vi "rawcdc_protocol.vi"() -> ()   [LabVIEW 2024]
doc: "This example performs writes and reads on a serial port, as directed by the user. You can press the Write and Read buttons, and change the Read Count, while the example is running.\n\nThe parameters set for the serial port must match the parameters of the connected instrument or device. In this example, the Read Count parameter specifies the number of bytes that the serial port reads. If there were more bytes at the port than the specified number, those bytes would not be read. If there were less bytes at the port than the specified number, you would receive a timeout error.\n\nThis example expands upon the flow control options for XON and XOFF, allowing the user to choose those control characters. Also, the user can enable or disable a termination character. Some devices require a termination character in order to identify the end of command strings. Some devices send a termination character to signify the end of data to be read. This example shows how you can end the Read operation once a termination character is detected in the buffer and/or append a termination character at the end of the Write data."
uses:
  <vilib>/Instr/_visa.llb/VISA Configure Serial Port (Instr).vi
panel:
  in  "Correction":dbl(slide) scale=-10.0..10.0
  out "Measured":dbl
  out "Waveform Chart":dbl[](graph)
  in  "Command List":string="stop\nencode 0\nslist 0 0\nsrate 6000\nps 2\ndec 1\ndeca 3\nnop\n\n\n"
  in  "Stop":bool
  in  "2108 CDC Virtual COM":refnum<visa-resource-name>="COM11"
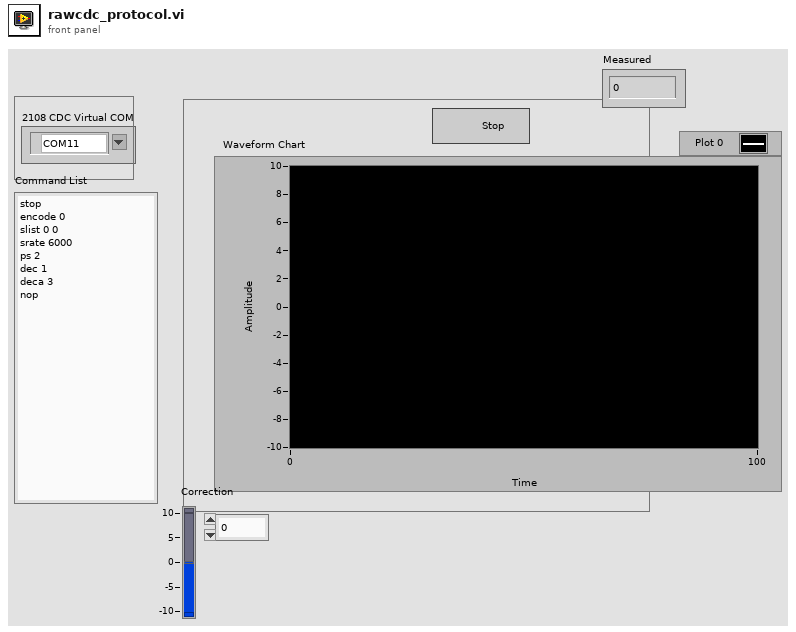
[diagram p1: front panel]
types:
  T1 = enum16{"big-endian, network order", "native, host order", "little-endian"}
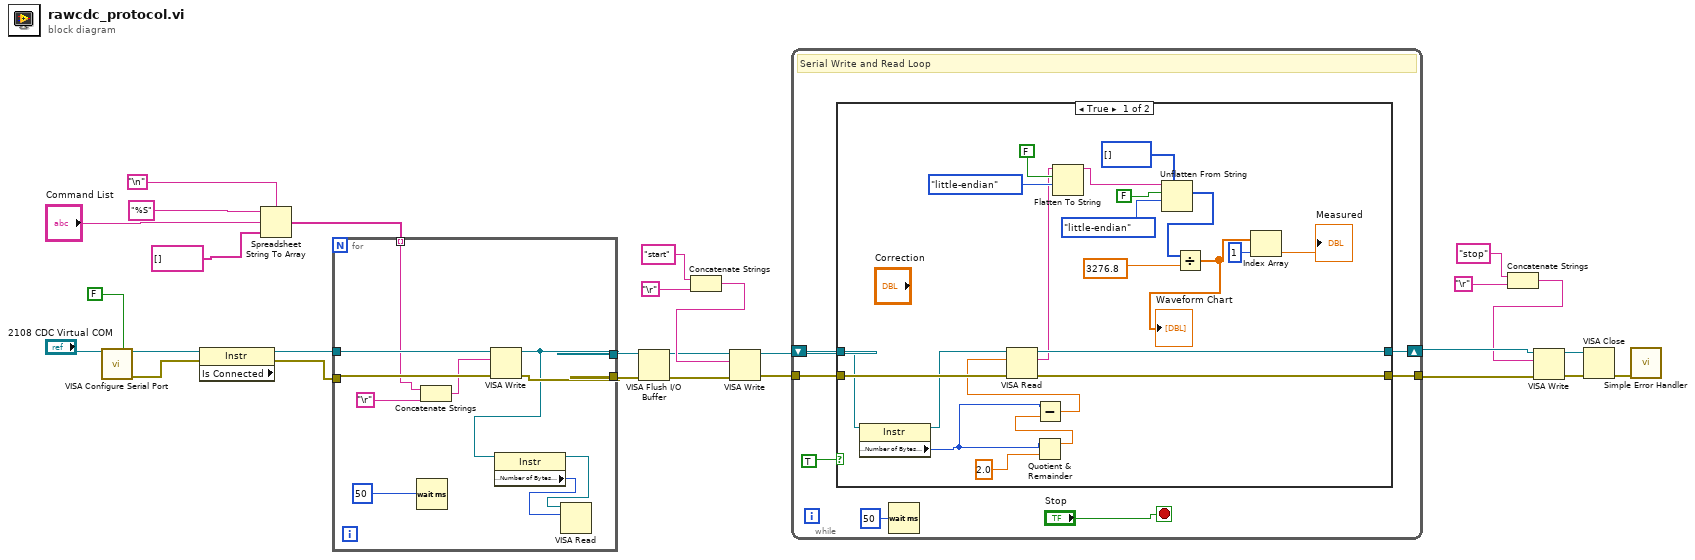
[diagram p0: block diagram]
diagram:
  n1 = call-poly "VISA Configure Serial Port"("VISA resource name"="2108 CDC Virtual COM", "Enable Termination\nChar (T)"=FALSE) -> ("VISA resource name out"=w26:refnum<visa-resource-name>, "error out"=w28:errorcluster)  [unwired: 8 in, 4 out]
  n2 = property class="Instr" props=["Is Connected"](reference=w26, error in=w28) -> (reference out=w2:refnum<visa-resource-name>, error out=w1:errorcluster)  [unwired: 1 out]
  n3 = Spreadsheet String To Array(delimiter (Tab)="\n", format string="%S", spreadsheet string="Command List", array type (2D Dbl)=string[] []) -> (array=w22:string[])
  n4 = for {
    tunnel: w22 -> [w35] mode=indexing
    tunnel: w2 -> [w38]
    tunnel: w1 -> [w37]
    tunnel: [w31] -> w6
    tunnel: [w32] -> w4
    n5 = Wait (ms)(milliseconds to wait=u32 50) -> ()  [unwired: 1 out]
    n6 = Concatenate Strings(w35, "\r") -> (w33:string)
    n7 = VISA Write(VISA resource name=w38, write buffer=w33, error in (no error)=w37) -> (VISA resource name out=w31:refnum<visa-resource-name>, error out=w32:errorcluster)  [unwired: 1 out]
    n8 = property class="Instr"(reference=w31) -> (reference out=w30:refnum<visa-resource-name>, "Serial Settings:Number of Bytes at Serial Port"=w29:u32)  [unwired: 1 in, 1 out]
    n9 = VISA Read(VISA resource name=w30, byte count=w29) -> ()  [unwired: 1 in, 4 out]
  }
  n10 = VISA Flush I/O Buffer(VISA resource name=w6, error in (no error)=w4) -> (VISA resource name out=w5:refnum<visa-resource-name>, error out=w3:errorcluster)  [unwired: 1 in]
  n11 = Concatenate Strings("start", "\r") -> (w10:string)
  n12 = VISA Write(VISA resource name=w5, write buffer=w10, error in (no error)=w3) -> (VISA resource name out=w9:refnum<visa-resource-name>, error out=w8:errorcluster)  [unwired: 1 out]
  n13 = while {
    shift-right: [w45] -> w19
    shift-left: w9 -> [w41]
    tunnel: w8 -> [w40]
    tunnel: [w43] -> w16
    stop <- "Stop" stop-if-true
    # "Serial Write and Read Loop"
    n14 = case shown="True" TRUE {
      tunnel: [w65 w68] -> w45
      tunnel: w41 -> [w63 w68]
      tunnel: w40 -> [w66 w67]
      tunnel: [w58 w67] -> w43
      frame True {
        n15 = property class="Instr"(reference=w63) -> (reference out=w57:refnum<visa-resource-name>, "Serial Settings:Number of Bytes at Serial Port"=w62:u32)  [unwired: 1 in, 1 out]
        n16 = Quotient & Remainder(x=w62, y=2.0) -> (x-y*floor(x/y)=w60:dbl)  [unwired: 1 out]
        n17 = Subtract(x=w62, y=w60) -> (x-y=w59:dbl)
        n18 = VISA Read(VISA resource name=w57, byte count=w59, error in (no error)=w66) -> (VISA resource name out=w65:refnum<visa-resource-name>, read buffer=w51:string, error out=w58:errorcluster)  [unwired: 1 out]
        n19 = Flatten To String(anything=w51, prepend array or string size? (T)=FALSE, byte order (0:big-endian, network order)=T1."little-endian") -> (data string=w52:string)  [unwired: 1 in, 2 out]
        n20 = Unflatten From String(type=i16[] [], binary string=w52, data includes array or string size? (T)=FALSE, byte order (0:big-endian, network order)=T1."little-endian") -> (value=w50:i16[])  [unwired: 1 in, 2 out]
        n21 = Divide(x=w50, y=3276.8) -> (x/y=w48:dbl[])
        "Waveform Chart" <- w48
        n22 = Index Array(array=w48, index=1) -> (element=→"Measured":dbl)
      }
      frame False {
      }
    }
    n23 = Wait (ms)(milliseconds to wait=u32 50) -> ()  [unwired: 1 out]
  }
  n24 = Concatenate Strings("stop", "\r") -> (w13:string)
  n25 = VISA Write(VISA resource name=w19, write buffer=w13, error in (no error)=w16) -> (VISA resource name out=w18:refnum<visa-resource-name>, error out=w17:errorcluster)  [unwired: 1 out]
  n26 = VISA Close(VISA resource name=w18, error in (no error)=w17) -> (error out=w27:errorcluster)
  n27 = call <vilib>:"Simple Error Handler.vi"("error in (no error)"=w27) -> ()  [unwired: 1 in, 8 out]
